vi "Dual XDCR Positioner.vi"(5 "Debug Mode?":bool, 6 "Initial Setup Complete":bool=TRUE, 7 "Main Digitizer":T1=enum."NI Digitizer", 8 "error in (no error)":errorcluster, 9 "Location":T2=enum."WCM Rotation", 10 "Dual XDCR Settings In":T3 {"XDCR Settings"."UT340 Controls"."Low Pass Filter (MHz)" min=-6 max=60 step=1; "XDCR Settings"."UT340 Controls"."High Pass Filter (MHz)" min=1 max=20 step=1; "XDCR Settings"."UT340 Controls"."Rep Rate (Hz)" min=20 step=1; "XDCR Settings"."UT340 Controls"."Pulse Width (ns)" min=100.0 max=250.0 step=2.0; "XDCR Settings"."UT340 Controls"."Voltage" min=100 max=250 step=2; "XDCR Settings"."UT340 Controls"."PC Gain (dB)" min=2 max=72; "XDCR Settings"."UT340 Controls"."PE Gain (dB)" min=-6 max=60 step=1; "XDCR Settings"."JSR Complete"."JSR Trigger Settings"."PRF (Hz)" items=["100 Hz"=0.1, "200 Hz"=0.2, "400 Hz"=0.4, "600 Hz"=0.6, "800 Hz"=0.8, "1000 Hz"=1.0, "1250 Hz"=1.25, "1500 Hz"=1.5, "1750 Hz"=1.75, "2000 Hz"=2.0, "2500 Hz"=2.5, "3000 Hz"=3.0, "3500 Hz"=3.5, "4000 Hz"=4.0, "4500 Hz"=4.5, "5000 Hz"=5.0]; "XDCR Settings"."JSR Complete"."JSR Trigger Settings"."Trigger Source" items=["Internal", "External"]; "XDCR Settings"."JSR Complete"."JSR Trigger Settings"."External Trigger Limit" items=["No Limit", "5 kHz"]; "XDCR Settings"."JSR Complete"."JSR Receive Settings"."Gain (dB)" min=-13 max=66 step=1; "XDCR Settings"."JSR Complete"."JSR Receive Settings"."Low Pass Filter" items=["5 MHz"=5, "10 MHz"=10, "15 MHz"=15, "22.5 MHz"=22, "35 MHz"=35, "50 MHz"=50]; "XDCR Settings"."JSR Complete"."JSR Receive Settings"."High Pass Filter" items=["DC"=0, "1 MHz"=1000, "2.5 MHz"=2500, "5 MHz"=5000, "7.5 MHz"=7500, "12.5 MHz"=12500]; "XDCR Settings"."JSR Complete"."JSR Receive Settings"."Receiver Mode" items=["Echo", "Through"]; "XDCR Settings"."JSR Complete"."JSR Pulse Settings"."Pulser Voltage (V)" items=["100"=100, "125"=125, "150"=150, "175"=175, "200"=200, "225"=225, "250"=250, "275"=275, "300"=300, "325"=325, "350"=350, "375"=375, "400"=400, "425"=425, "450"=450, "475"=475]; "XDCR Settings"."JSR Complete"."JSR Pulse Settings"."Pulser Impedance" items=["High z", "Low z"]; "XDCR Settings"."JSR Complete"."JSR Pulse Settings"."Pulse Energy Level" items=["0 (Minimum)", "1", "2", "3 (Maximum)"]; "XDCR Settings"."JSR Complete"."JSR Pulse Settings"."Damping" items=["331 Ohms"=331, "198 Ohms"=198, "142 Ohms"=142, "110 Ohms"=110, "92 Ohms"=92, "77 Ohms"=77, "67 Ohms"=67, "59 Ohms"=59, "52 Ohms"=52, "47 Ohms"=47, "43 Ohms"=43, "39 Ohms"=39, "37 Ohms"=37, "34 Ohms"=34, "32 Ohms"=32, "30 Ohms"=30]; "XDCR Settings"."Panametrics Settings"."FINE ATTENUATION" items=["00.0", "00.5", "01.0", "01.5", "02.0", "02.5", "03.0", "03.5", "04.0", "04.5", "05.0", "05.5", "06.0", "06.5", "07.0", "07.5", "08.0", "08.5", "09.0", "09.5", "10.0", "10.5", "11.0", "11.5", "12.0", "12.5", "13.0", "13.5", "14.0", "14.5", "15.0", "15.5"]; "XDCR Settings"."Panametrics Settings"."COARSE ATTENUATION" items=["00.0", "10.0", "20.0", "30.0", "40.0", "50.0"]; "XDCR Settings"."Panametrics Settings"."GAIN (db)" items=["26.0", "40.0", "54.0"]; "XDCR Settings"."Panametrics Settings"."PRF (KHz)" items=["XREMT", "EXBNC", "0.200", "0.500", "1.000", "2.000", "5.000", "10.00", "20.00"]; "XDCR Settings"."Panametrics Settings"."MODE" items=["P/ E", "THRU", "RPP", "EXT_PLSR"]; "XDCR Settings"."Panametrics Settings"."LP FILT (MHz)" items=["20", "50", "100", "200"]; "XDCR Settings"."Panametrics Settings"."HP FILT (KHz)" items=["1", "1000", "3000", "10000"]; "XDCR Settings"."Panametrics Settings"."DAMPING (Ohm)" items=["7", "10", "16", "20", "26", "30", "40", "50"]; "XDCR Settings"."Panametrics Settings"."ENERGY (uJ)" items=["1", "2", "4", "8", "16", "32"]; "XDCR Settings"."Daxsonics Settings"."Freq (MHz)" items=["4"=4, "5"=5, "6"=6, "8"=8, "10"=10, "12"=12, "14"=14, "15"=15, "16"=16, "17"=17, "18"=18, "20"=20, "25"=25, "30"=30, "35"=35, "40"=40, "45"=45, "50"=50]; "XDCR Settings"."Daxsonics Settings"."Voltage (V)" items=["0"=0, "5"=5, "10"=10, "15"=15, "20"=20, "25"=25, "30"=30, "35"=35, "40"=40, "45"=45, "50"=50, "55"=55, "60"=60, "65"=65, "70"=70, "75"=75, "80"=80, "85"=85, "90"=90, "95"=95, "100"=100, "110"=110, "120"=120, "130"=130, "140"=140, "150"=150, "160"=160, "170"=170, "180"=180, "190"=190]; "XDCR Settings"."Daxsonics Settings"."Gain (dB)" items=["22"=22, "25"=25, "28"=28, "31"=31, "34"=34, "37"=37, "40"=40, "43"=43, "46"=46, "49"=49, "52"=52, "55"=55, "58"=58, "61"=61, "64"=64, "67"=67]; "XDCR Settings"."Digitizer Settings"."Additional dig delay (ms)" format="%.2f"; "XDCR Settings"."Digitizer Settings"."Time scale per Div" items=["100 ns"=0.1, "200 ns"=0.2, "500 ns"=0.5, "1 micros"=1.0, "2 micros"=2.0, "5 micros"=5.0, "10 micros"=10.0, "20 micros"=20.0, "50 micros"=50.0, "100 micros"=100.0, "200 micros"=200.0, "500 micros"=500.0, "1 ms"=1000.0, "2 ms"=2000.0, "5 ms"=5000.0, "10 ms"=10000.0, "20 ms"=20000.0, "50 ms"=50000.0, "100 ms"=100000.0, "200 ms"=200000.0]; "XDCR Settings"."Digitizer Settings"."RF data Sampling"."rf points per line" min=1; "XDCR Settings"."Digitizer Settings"."RF data Sampling"."Ref Delay (ms)" format="%.2f"}, 11 "Motion Settings":T23={"No Motion?"=FALSE, "Motion System"=enum."NI 735x", "Motion Bd ID"=1, "Motion Profile"="SMAC1", "# Axis"=1, "Reverse Z axis?"=TRUE, "SMAC Axis"=0, "scan pair"=enum."y-(x) scan", "RT fps"=6.0, "Steps per mm"=[1000, 1000, 1000, 1000], "Motor Parameters"={"velocity ct/s"=[10000.0, 10000.0, 10000.0, 50000.0], "accel ct/s^2"=[50000.0, 50000.0, 50000.0, 200000.0]}, "One Way Scan"=FALSE, "Reverse One Way Scan"=FALSE, "Global Position (mm)"=[], "Plane"=0, "Distance between\nscan lines (um)"=0.0, "Distance between\nscan planes (um)"=0.0, "number of scan planes"=1, "Total steps in line"=0, "Xtra plane\ndistance  (um)"=100, "Xtra planes "=1, "Add Axis"=FALSE, "overshoot cts"=200, "BKPT Shift"=0, "Scan Start Time (ms)"=0, "ESP VISA"="GPIB::1::INSTR", "3rd Axis"=1, "GL Ref Out"=refnum, "Galil Address"=""} {"3rd Axis" items=["x", "y", "z", "w"]; "Xtra planes" min=1; "Xtra plane\ndistance  (um)" min=0; "Distance between\nscan planes (um)" format="%.2f"; "Distance between\nscan lines (um)" format="%.2f"; "SMAC Axis" items=["None"=0, "Axis 1"=1, "Axis 2"=2, "Axis 3"=3, "Axis 4"=4, "Axis 5"=5, "Axis 6"=6, "Axis 7"=7, "Axis 8"=8, "Vector Space 1"=17, "Vector Space 2"=18, "Vector Space 3"=19, "Vector Space 4"=20]; "Motion Bd ID" min=1 max=32 step=1}) -> (0 "error out":errorcluster, 1 "Switch T/R":u32, 2 "Dual XDCR Settings":T3 {"XDCR Settings"."UT340 Controls"."Low Pass Filter (MHz)" min=-6 max=60 step=1; "XDCR Settings"."UT340 Controls"."High Pass Filter (MHz)" min=1 max=20 step=1; "XDCR Settings"."UT340 Controls"."Rep Rate (Hz)" min=20 step=1; "XDCR Settings"."UT340 Controls"."Pulse Width (ns)" min=100.0 max=250.0 step=2.0; "XDCR Settings"."UT340 Controls"."Voltage" min=100 max=250 step=2; "XDCR Settings"."UT340 Controls"."PC Gain (dB)" min=2 max=72; "XDCR Settings"."UT340 Controls"."PE Gain (dB)" min=-6 max=60 step=1; "XDCR Settings"."JSR Complete"."JSR Trigger Settings"."PRF (Hz)" items=["100 Hz"=0.1, "200 Hz"=0.2, "400 Hz"=0.4, "600 Hz"=0.6, "800 Hz"=0.8, "1000 Hz"=1.0, "1250 Hz"=1.25, "1500 Hz"=1.5, "1750 Hz"=1.75, "2000 Hz"=2.0, "2500 Hz"=2.5, "3000 Hz"=3.0, "3500 Hz"=3.5, "4000 Hz"=4.0, "4500 Hz"=4.5, "5000 Hz"=5.0]; "XDCR Settings"."JSR Complete"."JSR Trigger Settings"."Trigger Source" items=["Internal", "External"]; "XDCR Settings"."JSR Complete"."JSR Trigger Settings"."External Trigger Limit" items=["No Limit", "5 kHz"]; "XDCR Settings"."JSR Complete"."JSR Receive Settings"."Gain (dB)" min=-13 max=66 step=1; "XDCR Settings"."JSR Complete"."JSR Receive Settings"."Low Pass Filter" items=["5 MHz"=5, "10 MHz"=10, "15 MHz"=15, "22.5 MHz"=22, "35 MHz"=35, "50 MHz"=50]; "XDCR Settings"."JSR Complete"."JSR Receive Settings"."High Pass Filter" items=["DC"=0, "1 MHz"=1000, "2.5 MHz"=2500, "5 MHz"=5000, "7.5 MHz"=7500, "12.5 MHz"=12500]; "XDCR Settings"."JSR Complete"."JSR Receive Settings"."Receiver Mode" items=["Echo", "Through"]; "XDCR Settings"."JSR Complete"."JSR Pulse Settings"."Pulser Voltage (V)" items=["100"=100, "125"=125, "150"=150, "175"=175, "200"=200, "225"=225, "250"=250, "275"=275, "300"=300, "325"=325, "350"=350, "375"=375, "400"=400, "425"=425, "450"=450, "475"=475]; "XDCR Settings"."JSR Complete"."JSR Pulse Settings"."Pulser Impedance" items=["High z", "Low z"]; "XDCR Settings"."JSR Complete"."JSR Pulse Settings"."Pulse Energy Level" items=["0 (Minimum)", "1", "2", "3 (Maximum)"]; "XDCR Settings"."JSR Complete"."JSR Pulse Settings"."Damping" items=["331 Ohms"=331, "198 Ohms"=198, "142 Ohms"=142, "110 Ohms"=110, "92 Ohms"=92, "77 Ohms"=77, "67 Ohms"=67, "59 Ohms"=59, "52 Ohms"=52, "47 Ohms"=47, "43 Ohms"=43, "39 Ohms"=39, "37 Ohms"=37, "34 Ohms"=34, "32 Ohms"=32, "30 Ohms"=30]; "XDCR Settings"."Panametrics Settings"."FINE ATTENUATION" items=["00.0", "00.5", "01.0", "01.5", "02.0", "02.5", "03.0", "03.5", "04.0", "04.5", "05.0", "05.5", "06.0", "06.5", "07.0", "07.5", "08.0", "08.5", "09.0", "09.5", "10.0", "10.5", "11.0", "11.5", "12.0", "12.5", "13.0", "13.5", "14.0", "14.5", "15.0", "15.5"]; "XDCR Settings"."Panametrics Settings"."COARSE ATTENUATION" items=["00.0", "10.0", "20.0", "30.0", "40.0", "50.0"]; "XDCR Settings"."Panametrics Settings"."GAIN (db)" items=["26.0", "40.0", "54.0"]; "XDCR Settings"."Panametrics Settings"."PRF (KHz)" items=["XREMT", "EXBNC", "0.200", "0.500", "1.000", "2.000", "5.000", "10.00", "20.00"]; "XDCR Settings"."Panametrics Settings"."MODE" items=["P/ E", "THRU", "RPP", "EXT_PLSR"]; "XDCR Settings"."Panametrics Settings"."LP FILT (MHz)" items=["20", "50", "100", "200"]; "XDCR Settings"."Panametrics Settings"."HP FILT (KHz)" items=["1", "1000", "3000", "10000"]; "XDCR Settings"."Panametrics Settings"."DAMPING (Ohm)" items=["7", "10", "16", "20", "26", "30", "40", "50"]; "XDCR Settings"."Panametrics Settings"."ENERGY (uJ)" items=["1", "2", "4", "8", "16", "32"]; "XDCR Settings"."Daxsonics Settings"."Freq (MHz)" items=["4"=4, "5"=5, "6"=6, "8"=8, "10"=10, "12"=12, "14"=14, "15"=15, "16"=16, "17"=17, "18"=18, "20"=20, "25"=25, "30"=30, "35"=35, "40"=40, "45"=45, "50"=50]; "XDCR Settings"."Daxsonics Settings"."Voltage (V)" items=["0"=0, "5"=5, "10"=10, "15"=15, "20"=20, "25"=25, "30"=30, "35"=35, "40"=40, "45"=45, "50"=50, "55"=55, "60"=60, "65"=65, "70"=70, "75"=75, "80"=80, "85"=85, "90"=90, "95"=95, "100"=100, "110"=110, "120"=120, "130"=130, "140"=140, "150"=150, "160"=160, "170"=170, "180"=180, "190"=190]; "XDCR Settings"."Daxsonics Settings"."Gain (dB)" items=["22"=22, "25"=25, "28"=28, "31"=31, "34"=34, "37"=37, "40"=40, "43"=43, "46"=46, "49"=49, "52"=52, "55"=55, "58"=58, "61"=61, "64"=64, "67"=67]; "XDCR Settings"."Digitizer Settings"."Additional dig delay (ms)" format="%.2f"; "XDCR Settings"."Digitizer Settings"."Time scale per Div" items=["100 ns"=0.1, "200 ns"=0.2, "500 ns"=0.5, "1 micros"=1.0, "2 micros"=2.0, "5 micros"=5.0, "10 micros"=10.0, "20 micros"=20.0, "50 micros"=50.0, "100 micros"=100.0, "200 micros"=200.0, "500 micros"=500.0, "1 ms"=1000.0, "2 ms"=2000.0, "5 ms"=5000.0, "10 ms"=10000.0, "20 ms"=20000.0, "50 ms"=50000.0, "100 ms"=100000.0, "200 ms"=200000.0]; "XDCR Settings"."Digitizer Settings"."RF data Sampling"."rf points per line" min=1; "XDCR Settings"."Digitizer Settings"."RF data Sampling"."Ref Delay (ms)" format="%.2f"}, 3 "Motion Settings Out":T23={"No Motion?"=FALSE, "Motion System"=enum."NI 735x", "Motion Bd ID"=1, "Motion Profile"="SMAC1", "# Axis"=1, "Reverse Z axis?"=TRUE, "SMAC Axis"=0, "scan pair"=enum."y-(x) scan", "RT fps"=6.0, "Steps per mm"=[1000, 1000, 1000, 1000], "Motor Parameters"={"velocity ct/s"=[10000.0, 10000.0, 10000.0, 50000.0], "accel ct/s^2"=[50000.0, 50000.0, 50000.0, 200000.0]}, "One Way Scan"=FALSE, "Reverse One Way Scan"=FALSE, "Global Position (mm)"=[], "Plane"=0, "Distance between\nscan lines (um)"=0.0, "Distance between\nscan planes (um)"=0.0, "number of scan planes"=1, "Total steps in line"=0, "Xtra plane\ndistance  (um)"=100, "Xtra planes "=1, "Add Axis"=FALSE, "overshoot cts"=200, "BKPT Shift"=0, "Scan Start Time (ms)"=0, "ESP VISA"="GPIB::1::INSTR", "3rd Axis"=1, "GL Ref Out"=refnum, "Galil Address"=""} {"3rd Axis" items=["x", "y", "z", "w"]; "Xtra planes" min=1; "Xtra plane\ndistance  (um)" min=0; "Distance between\nscan planes (um)" format="%.2f"; "Distance between\nscan lines (um)" format="%.2f"; "SMAC Axis" items=["None"=0, "Axis 1"=1, "Axis 2"=2, "Axis 3"=3, "Axis 4"=4, "Axis 5"=5, "Axis 6"=6, "Axis 7"=7, "Axis 8"=8, "Vector Space 1"=17, "Vector Space 2"=18, "Vector Space 3"=19, "Vector Space 4"=20]; "Motion Bd ID" min=1 max=32 step=1}, 4 "Default Selected?":bool)   [LabVIEW 2022 SP3]
uses:
  Motion Controllers/NI_controller/-NI_MotionRoutines/MotionParameters.ctl
  Motion Controllers/NI_controller/-NI_MotionRoutines/MotionSys.ctl
  Motion Controllers/-MotionRoutines/ScanAxis.ctl
  Motion Controllers/-MotionRoutines/3rdAxis.ctl
  Dual XDCR Complete Settings.ctl
  XDCRSettings.ctl
  Pulsers/Daxsonics/-DaxSubroutines/Dax_Control_Cluster.ctl
  Pulsers/Panametrics/Pana5900.ctl
  Pulsers/JSR/Controls/JSR Complete.ctl
  Pulsers/JSR/Controls/JSR Pulse.ctl
  Pulsers/JSR/Controls/Damping.ctl
  Pulsers/JSR/Controls/Energy.ctl
  Pulsers/JSR/Controls/Z.ctl
  Pulsers/JSR/Controls/Volt.ctl
  Pulsers/JSR/Controls/JSR Recieve.ctl
  Pulsers/JSR/Controls/Mode.ctl
  Pulsers/JSR/Controls/HPF.ctl
  Pulsers/JSR/Controls/LPF.ctl
  Pulsers/JSR/Controls/Gain.ctl
  Pulsers/JSR/Controls/JSR Trigger.ctl
  Pulsers/JSR/Controls/Trig Limit.ctl
  Pulsers/JSR/Controls/Trig Source.ctl
  Pulsers/JSR/Controls/PRF.ctl
  Pulsers/UTEX/Controls/UTEX Controls.ctl
  -ScanSystem/Controls/location.ctl
  Digitizers/-DigitizerRoutines/Digitizer.ctl
  <vilib>/Motion/FlexMotion/CustomControls/CustomControls.llb/AxisOrVectorSpaceControl To Control.flx
panel:
  out "Abort":bool
  # "1-D and 2-D B scan settings"
  # "1-D and 2-D B scan settings"
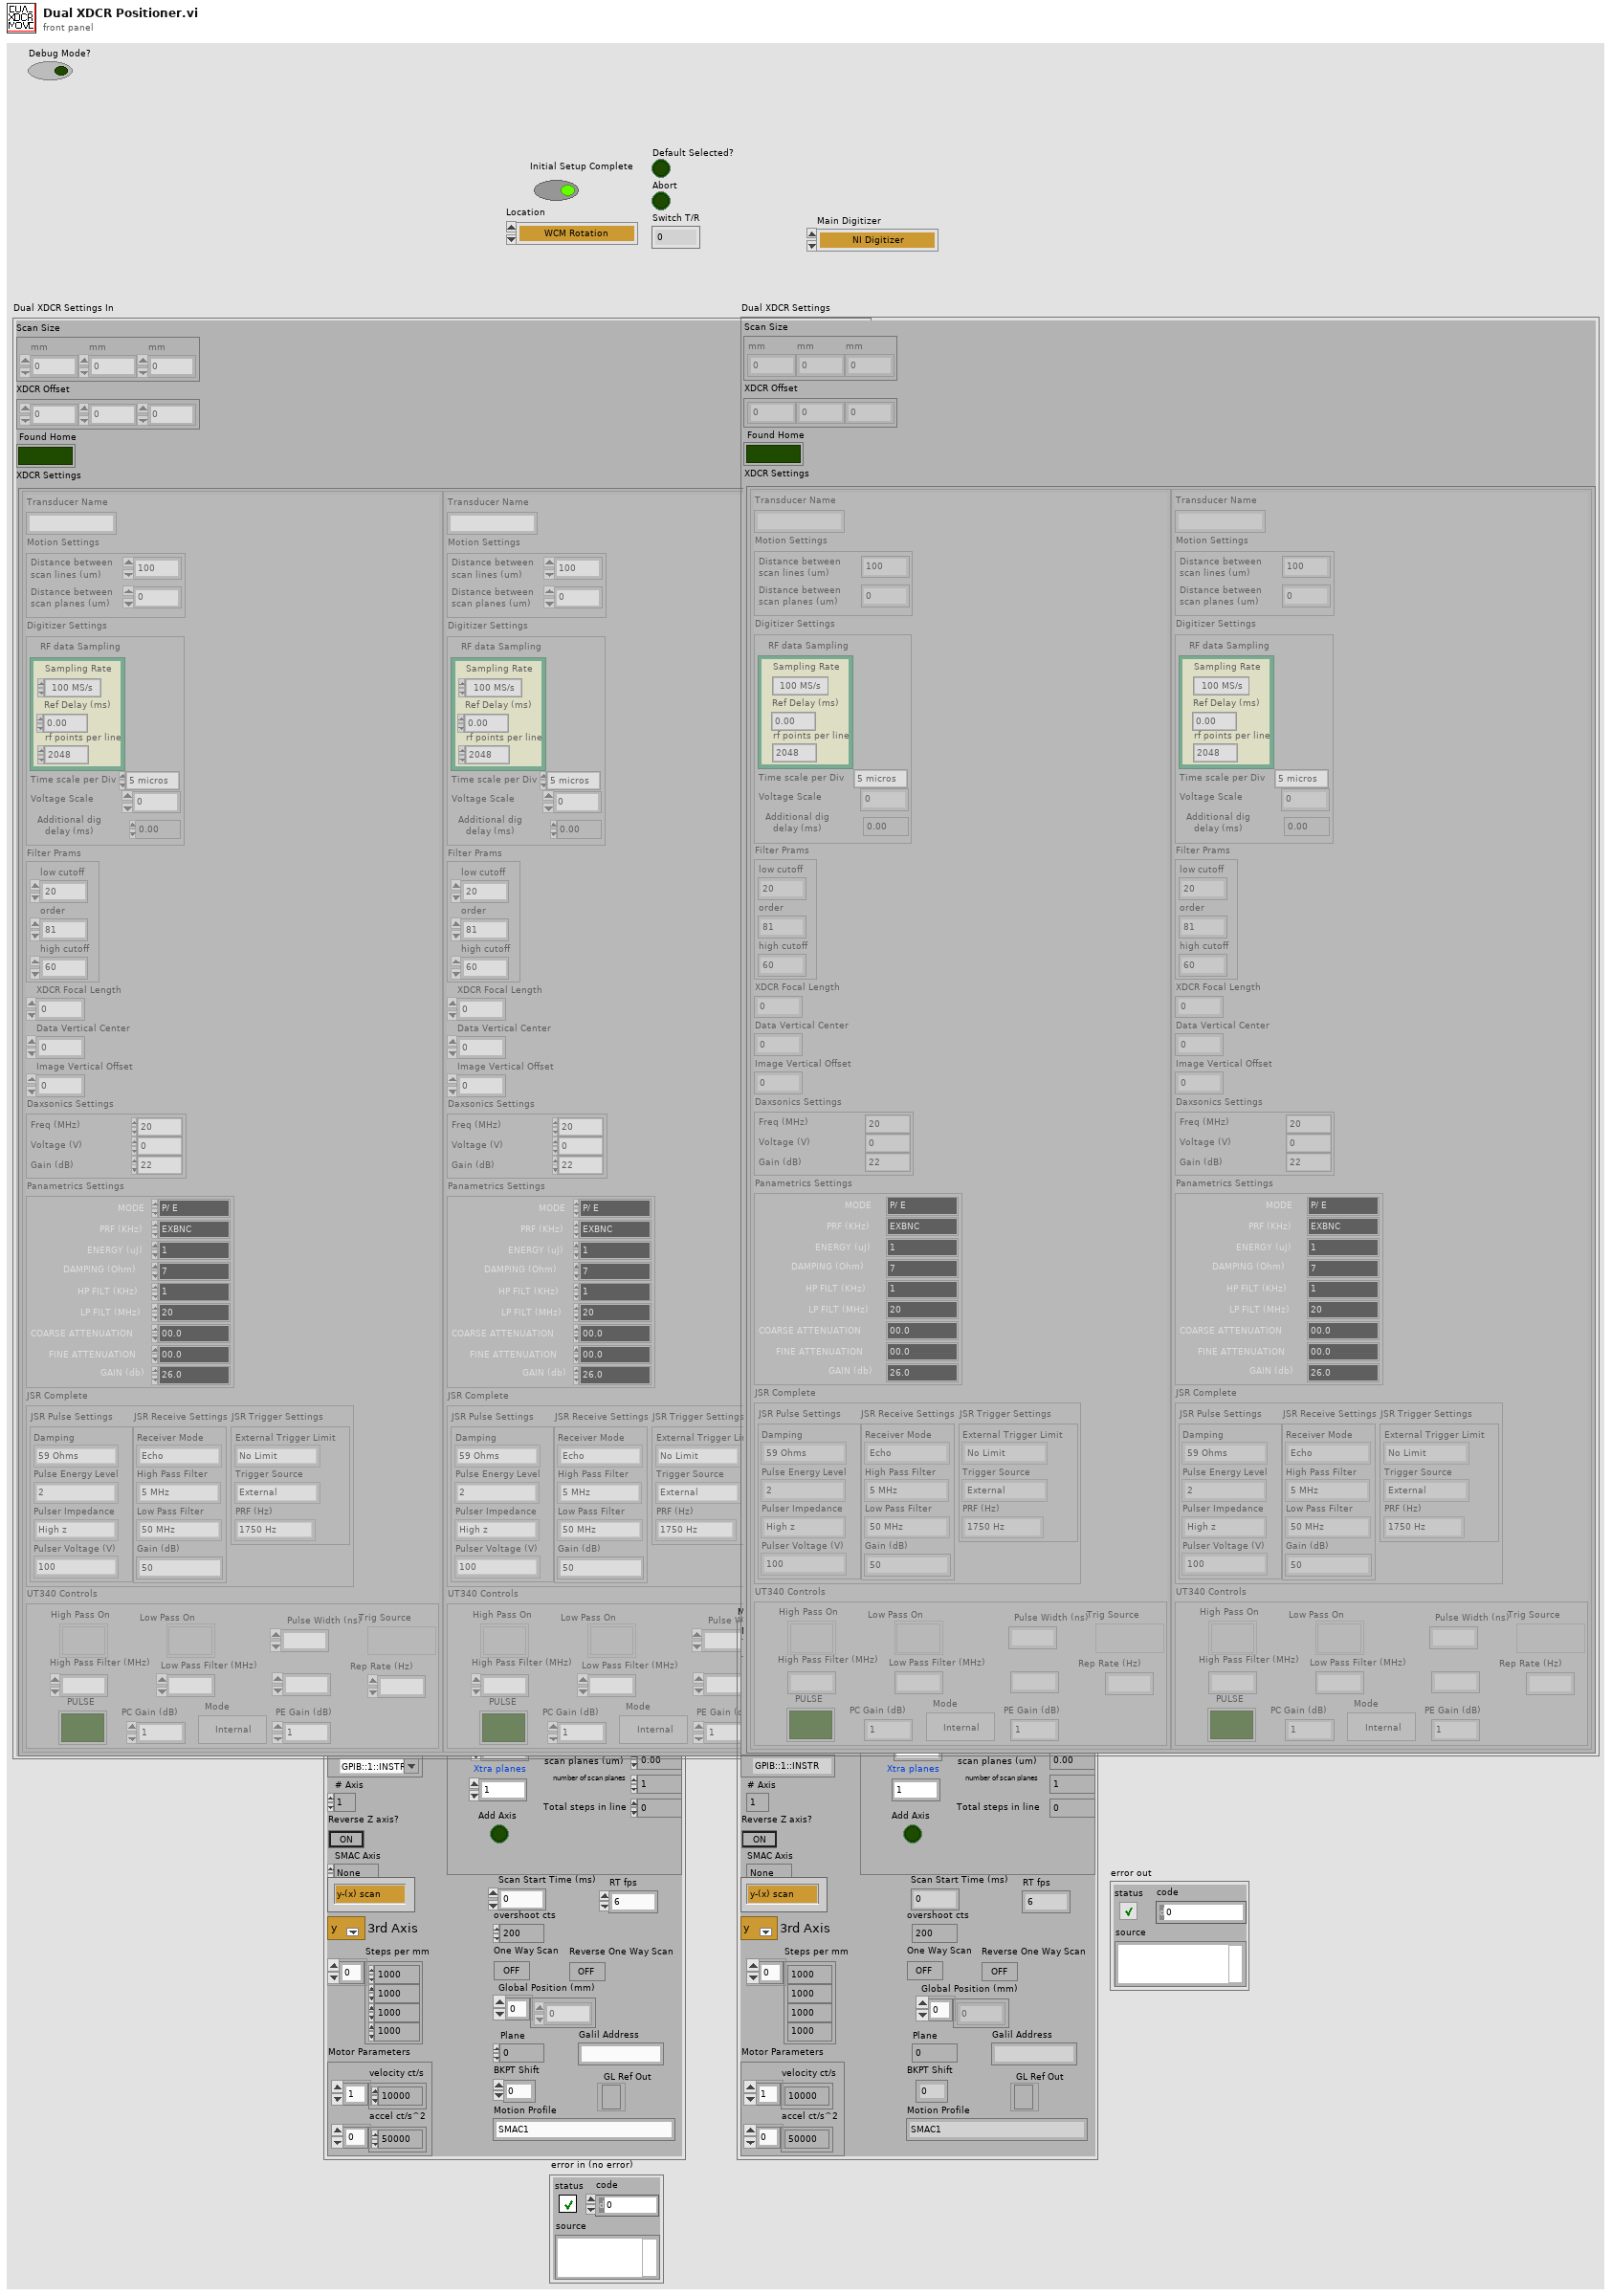
[diagram p1: front panel]
types:
  T1 = typedef "Digitizer.ctl" = enum16{"Acqiris Digitizer", "NI Digitizer", "LeCroy", "GaGe", "AlazarTech", "No Digitizer", "Teledyne"}
  T2 = typedef "location.ctl" = enum16{"Automatic", "WCM Main", "Hawaii", "Columbia MM3000", "Columbia  NI System", "NYU", "RRI 2", "UHI Allen", "CUMC RT", "Chiba", "Stony Brook", "WCM Microscopy", "WCM Aeoretch", "WCM Optics Lab", "WCM Main 2Axis", "WCM Rotation", "WCM SAM SMAC", "SERI GP"}
  T3 = typedef "Dual XDCR Complete Settings.ctl" = cluster{"Scan Size":dbl[], "XDCR Offset":dbl[], "Found Home":bool, "XDCR Settings":T4[]}
  T4 = typedef "XDCRSettings.ctl" = cluster{"Transducer Name":string, "Motion Settings":cluster{"Distance between\nscan lines (um)":sgl, "Distance between\nscan planes (um)":sgl}, "Digitizer Settings":cluster{"RF data Sampling":cluster{"Sampling Rate":dbl, "Ref Delay (ms)":dbl, "rf points per line":i32}, "Time scale per Div":dbl, "Voltage Scale":dbl, "Additional dig delay (ms)":dbl}, "Filter Prams":cluster{"low cutoff":i32, "order":i32, "high cutoff":i32}, "XDCR Focal Length":dbl, "Data Vertical Center":dbl, "Image Vertical Offset":dbl, "Daxsonics Settings":T5, "Panametrics Settings":T6, "JSR Complete":T7, "UT340 Controls":T22}
  T5 = typedef "Dax_Control_Cluster.ctl" = cluster{"Freq (MHz) ":u16, "Voltage (V)":u16, "Gain (dB)":u16}
  T6 = typedef "Pana5900.ctl" = cluster{"ENERGY (uJ)":u16, "DAMPING (Ohm)":u16, "HP FILT (KHz) ":u16, "LP FILT (MHz)":u16, "MODE":u16, "PRF (KHz)":u16, "GAIN (db)":u16, "COARSE ATTENUATION":u16, "FINE ATTENUATION":u16}
  T7 = typedef "JSR Complete.ctl" = cluster{"JSR Pulse Settings":T8, "JSR Receive Settings":T13, "JSR Trigger Settings":T18}
  T8 = typedef "JSR Pulse.ctl" = cluster{"Damping":T9, "Pulse Energy Level":T10, "Pulser Impedance":T11, "Pulser Voltage (V)":T12}
  T9 = typedef "Damping.ctl" = i16
  T10 = typedef "Energy.ctl" = u16
  T11 = typedef "Z.ctl" = u16
  T12 = typedef "Volt.ctl" = i16
  T13 = typedef "JSR Recieve.ctl" = cluster{"Receiver Mode":T14, "High Pass Filter":T15, "Low Pass Filter":T16, "Gain (dB)":T17}
  T14 = typedef "Mode.ctl" = i8
  T15 = typedef "HPF.ctl" = u16
  T16 = typedef "LPF.ctl" = u16
  T17 = typedef "Gain.ctl" = i8
  T18 = typedef "JSR Trigger.ctl" = cluster{"External Trigger Limit":T19, "Trigger Source":T20, "PRF (Hz)":T21}
  T19 = typedef "Trig Limit.ctl" = i8
  T20 = typedef "Trig Source.ctl" = i8
  T21 = typedef "PRF.ctl" = dbl
  T22 = typedef "UTEX Controls.ctl" = cluster{"High Pass On":bool, "High Pass Filter (MHz)":i16, "Low Pass On":bool, "Low Pass Filter (MHz)":i16, "PE Gain (dB)":i16, "Voltage":i16, "Pulse Width (ns)":dbl, "Mode":bool, "PC Gain (dB)":i16, "Trig Source":bool, "Rep Rate (Hz)":i16, "PULSE":bool}
  T23 = typedef "MotionParameters.ctl" = cluster{"No Motion?":bool, "Motion System":T24, "Motion Bd ID":u8, "Motion Profile":string, "# Axis":i8, "Reverse Z axis?":bool, "SMAC Axis":u16, "scan pair":T25, "RT fps":sgl, "Steps per mm":i32[], "Motor Parameters":cluster{"velocity ct/s":dbl[], "accel ct/s^2":dbl[]}, "One Way Scan":bool, "Reverse One Way Scan":bool, "Global Position (mm)":dbl[], "Plane":i32, "Distance between\nscan lines (um)":sgl, "Distance between\nscan planes (um)":sgl, "number of scan planes":i32, "Total steps in line":i32, "Xtra plane\ndistance  (um)":i32, "Xtra planes ":i32, "Add Axis":bool, "overshoot cts":i32, "BKPT Shift":i32, "Scan Start Time (ms)":u32, "ESP VISA":refnum<visa-resource-name>, "3rd Axis":T26, "GL Ref Out":refnum<k7>, "Galil Address":string}
  T24 = typedef "MotionSys.ctl" = enum16{"MM3000", "NI 735x", "Newport ESP", "No Motion Card", "Galil"}
  T25 = typedef "ScanAxis.ctl" = enum16{"y-(x) scan", "x-(y) scan", "z-(x) scan", "z-(y) scan", "y-(z) scan", "x-(z) scan", "w-(x) scan", "w-(y) scan", "w-(z) scan", "x-(w) scan", "y-(w) scan", "z-(w) scan"}
  T26 = typedef "3rdAxis.ctl" = u16
  T27 = enum16{"Left Button", "Center Button", "Right Button", "Window Close"}
  T28 = cluster{"1":bool, "2":bool, "3":bool, "4":bool, "5":bool, "6":bool, "7":bool, "8":bool}
  T29 = enum16{"Absolute Position", "Relative Position", "Velocity", "Relative to Cap Pos", "Modulus Position", "Absolute Contouring", "Relative Contouring"}
  T30 = enum16{"Home", "Index", "Center", "Forward Limit", "Reverse Limit", "Run Sequence"}
  T31 = typedef "AxisOrVectorSpaceControl To Control.flx" = u16
  T32 = typedef "Bd Id Out" = u8
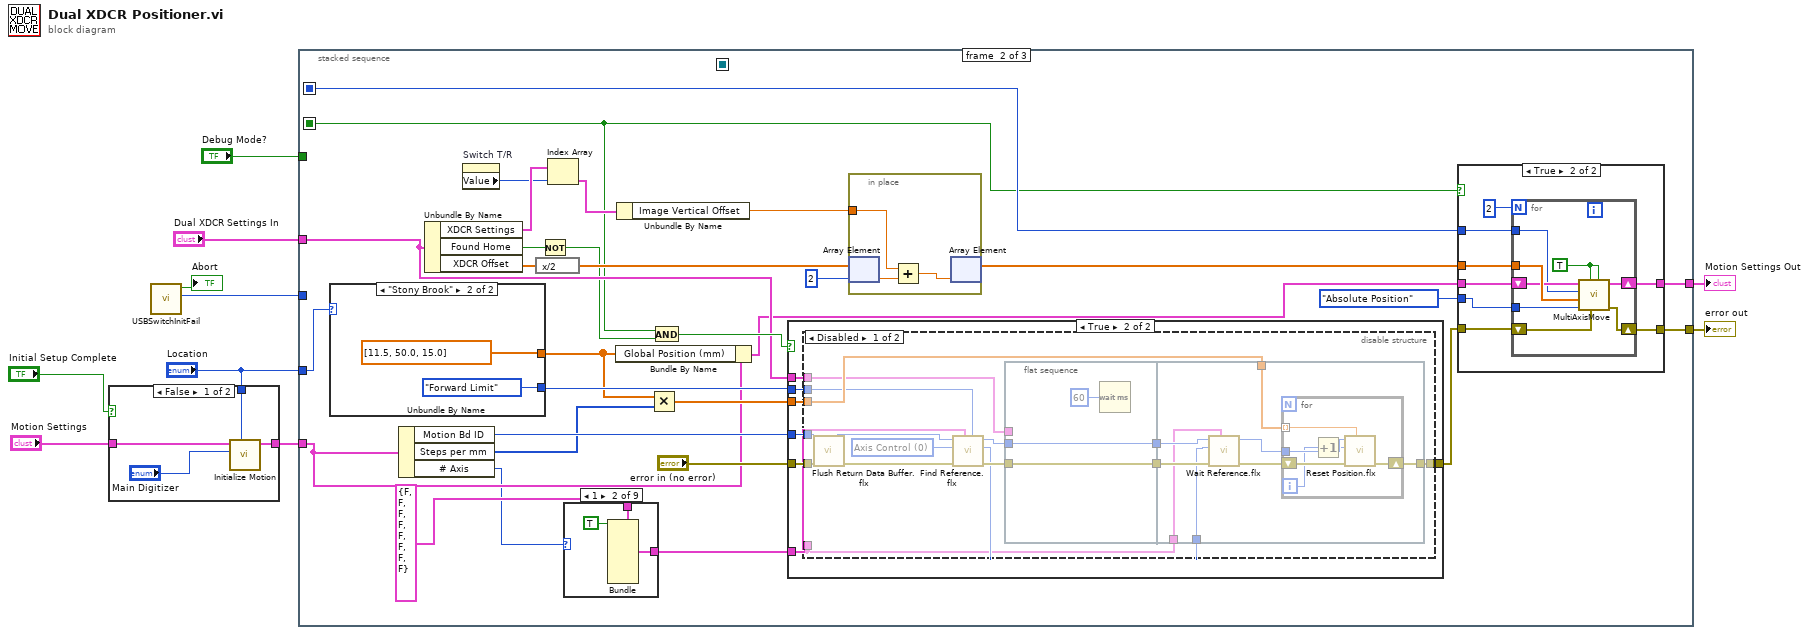
[diagram p0: block diagram]
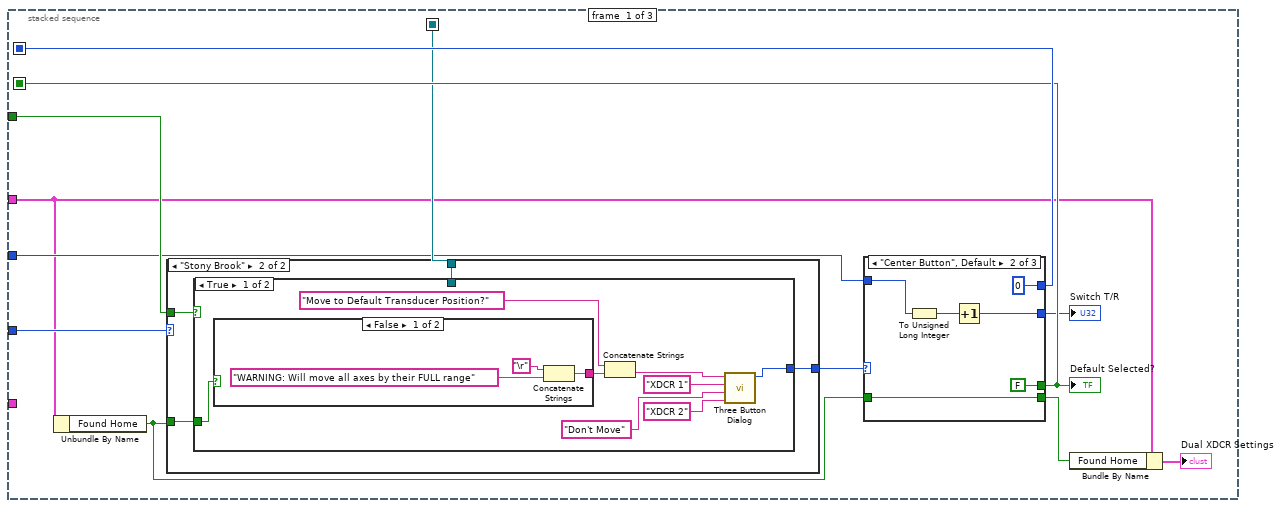
[diagram p3: hidden frame]
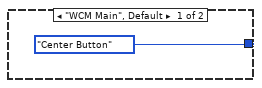
[diagram p4: hidden frame]
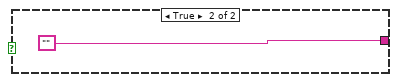
[diagram p5: hidden frame]
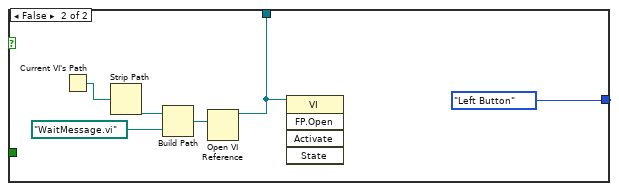
[diagram p6: hidden frame]
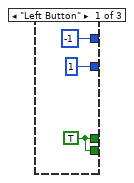
[diagram p7: hidden frame]
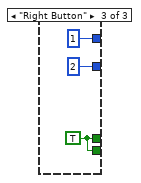
[diagram p8: hidden frame]
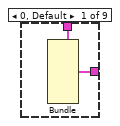
[diagram p9: hidden frame]
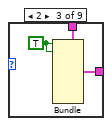
[diagram p10: hidden frame]
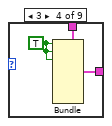
[diagram p11: hidden frame]
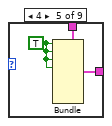
[diagram p12: hidden frame]
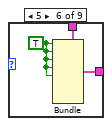
[diagram p13: hidden frame]
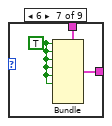
[diagram p14: hidden frame]
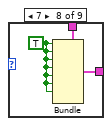
[diagram p15: hidden frame]
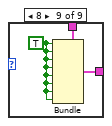
[diagram p16: hidden frame]
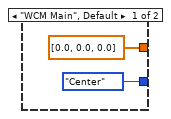
[diagram p20: hidden frame]
diagram:
  n1 = case shown="False" "Initial Setup Complete" {
    tunnel: "Motion Settings" -> [w14 w15]
    tunnel: [w13 w15] -> w6
    tunnel: "Location" -> [w11 _]
    frame False {
      n2 = call "Initialize Motion.vi"("Location"=w11, "Main Digitizer"="Main Digitizer", "Motion Settings In"=w14) -> ("Motion Settings"=w13:T23)  [unwired: 6 in, 2 out]
    }
    frame True {
    }
  }
  n3 = call "USBSwitchInitFail.vi"() -> ("Transducer"=w2:enum16{"Transducer 1", "Transducer 2"}, "Abort"=→"Abort":bool)  [unwired: 10 in]
  n4 = stacked-sequence {
    seq-local: [w24 _ _] -> [_ w84 w184]
    seq-local: [w23 _ _] -> [_ w67 _]
    seq-local: [w19 _ _] -> [_ _ w185]
    tunnel: "Dual XDCR Settings In" -> [w16 w81 _]
    tunnel: [_ w83 _] -> w9
    tunnel: [_ w82 _] -> w8
    tunnel: w6 -> [_ w79 _]
    tunnel: "Location" -> [w22 w69 w186]
    tunnel: "Debug Mode?" -> [w18 _ _]
    tunnel: w2 -> [w17 _ _]
    frame #0 {
      n5 = Unbundle By Name(w16) -> ("Found Home"=w21:bool)
      n6 = case shown="\"Stony Brook\"" w22 {
        tunnel: [T27."Center Button" ("Which Button?") w32] -> w27
        tunnel: w21 -> [_ w30]
        tunnel: [_ w31] -> w19
        tunnel: w18 -> [_ w29]
        frame "WCM Main", Default {
        }
        frame "Stony Brook" {
          n7 = case shown="True" w29 {
            tunnel: [w34 T27."Left Button" ("Which Button?")] -> w32
            tunnel: [_ w49] -> w31
            tunnel: w30 -> [w33 _]
            frame True {
              n8 = case shown="False" w33 {
                tunnel: [w41 "" ("message")] -> w35
                frame False {
                  n9 = Concatenate Strings("\r", "WARNING: Will move all axes by their FULL range" ("message")) -> (w41:string)
                }
                frame True {
                }
              }
              n10 = Concatenate Strings("Move to Default Transducer Position?" ("message"), w35) -> (w37:string)
              n11 = call <vilib>:"Three Button Dialog.vi"("Right Button Text (\"Cancel\")"="XDCR 2" ("Right Button Text (\"Cancel\")"), "Center Button Text (\"No\")"="Don't Move" ("F button name (\"Cancel\")"), "Left Button Text (\"Yes\")"="XDCR 1" ("T button name (\"OK\")"), "message"=w37) -> ("Which Button?"=w34:T27)  [unwired: 7 in]
            }
            frame False {
              n12 = Current VI's Path() -> (path=w47:path)
              n13 = Strip Path(path=w47) -> (stripped path=w45:path)  [unwired: 1 out]
              n14 = Build Path(base path=w45, name or relative path=path "WaitMessage.vi" ("vi path")) -> (appended path=w48:path)
              n15 = Open VI Reference(vi path=w48) -> (vi reference=w49:refnum<vi>)  [unwired: 5 in, 1 out]
              n16 = invoke class="VI" method="FP.Open"(reference=w49) -> ()  [unwired: 4 in, 5 out]
            }
          }
        }
      }
      n17 = case shown="\"Center Button\", Default" w27 {
        tunnel: [w51 FALSE w60] -> w23
        tunnel: [-1 ("Move Polarity") 0 ("Move Polarity") 1 ("Move Polarity")] -> w24
        tunnel: [u32 1 ("Switch T/R") w57 u32 2 ("Switch T/R")] -> w20
        tunnel: [w51 w56 w60] -> w26
        tunnel: w21 -> [_ w56 _]
        tunnel: w17 -> [_ w54 _]
        frame "Left Button" {
          w51 = TRUE ("Found Home")
        }
        frame "Center Button", Default {
          n18 = To Unsigned Long Integer(number=w54) -> (unsigned 32bit integer=w55:u32)
          n19 = Increment(x=w55) -> (x+1=w57:u32)
        }
        frame "Right Button" {
          w60 = TRUE ("Found Home")
        }
      }
      "Switch T/R" <- w20
      "Default Selected?" <- w23
      n20 = Bundle By Name(cluster=w16, "Found Home"=w26) -> (→"Dual XDCR Settings":T3)
    }
    frame #1 {
      n21 = case shown="\"Stony Brook\"" w69 {
        tunnel: [T30."Center" ("Search Type") T30."Forward Limit" ("Search Type")] -> w89
        tunnel: [dbl[] [0.0, 0.0, 0.0] ("Primary Reset Position (0)") dbl[] [11.5, 50.0, 15.0] ("Primary Reset Position (0)")] -> w78
        frame "WCM Main", Default {
        }
        frame "Stony Brook" {
        }
      }
      n22 = Unbundle By Name(w79) -> ("Motion Bd ID"=w88:u8, "Steps per mm"=w77:i32[], "# Axis"=w63:i8)
      n23 = Unbundle By Name(w81) -> ("XDCR Settings"=w76:T4[], "Found Home"=w87:bool, "XDCR Offset"=w85:dbl[])
      n24 = property on="Switch T/R" class="DigNum (strict)"() -> ("Value"=w75:u32)  [unwired: 2 in, 2 out]
      n25 = expression code="x/2"(w85) -> (w73:dbl[])
      n26 = Not(x=w87) -> (.not. x?=w66:bool)
      n27 = Index Array(array=w76, index=w75) -> (element=w74:T4)
      n28 = case shown="1" w63 {
        tunnel: [w94 w97 w100 w103 w106 w109 w112 w115 w118] -> w65
        tunnel: T28 {"1"=FALSE, "2"=FALSE, "3"=FALSE, "4"=FALSE, "5"=FALSE, "6"=FALSE, "7"=FALSE, "8"=FALSE} ("Axis/VS Map (Disabled)") -> [w93 w96 w99 w102 w105 w108 w111 w114 w117]
        frame 0, Default {
          n29 = Bundle(cluster=w93) -> (w94:T28)  [unwired: 8 in]
        }
        frame 1 {
          n30 = Bundle(cluster=w96, "1"=TRUE) -> (w97:T28)  [unwired: 7 in]
        }
        frame 2 {
          w98 = TRUE ("1")
          n31 = Bundle(cluster=w99, "1"=w98, "2"=w98) -> (w100:T28)  [unwired: 6 in]
        }
        frame 3 {
          w101 = TRUE ("1")
          n32 = Bundle(cluster=w102, "1"=w101, "2"=w101, "3"=w101) -> (w103:T28)  [unwired: 5 in]
        }
        frame 4 {
          w104 = TRUE ("1")
          n33 = Bundle(cluster=w105, "1"=w104, "2"=w104, "3"=w104, "4"=w104) -> (w106:T28)  [unwired: 4 in]
        }
        frame 5 {
          w107 = TRUE ("1")
          n34 = Bundle(cluster=w108, "1"=w107, "2"=w107, "3"=w107, "4"=w107, "5"=w107) -> (w109:T28)  [unwired: 3 in]
        }
        frame 6 {
          w110 = TRUE ("1")
          n35 = Bundle(cluster=w111, "1"=w110, "2"=w110, "3"=w110, "4"=w110, "5"=w110, "6"=w110) -> (w112:T28)  [unwired: 2 in]
        }
        frame 7 {
          w113 = TRUE ("1")
          n36 = Bundle(cluster=w114, "1"=w113, "2"=w113, "3"=w113, "4"=w113, "5"=w113, "6"=w113, "7"=w113) -> (w115:T28)  [unwired: 1 in]
        }
        frame 8 {
          w116 = TRUE ("1")
          n37 = Bundle(cluster=w117, "1"=w116, "2"=w116, "3"=w116, "4"=w116, "5"=w116, "6"=w116, "7"=w116, "8"=w116) -> (w118:T28)
        }
      }
      n38 = Bundle By Name(cluster=w79, "Global Position (mm)"=w78) -> (w80:T23)
      n39 = Unbundle By Name(w74) -> ("Image Vertical Offset"=w71:dbl)
      n40 = Multiply(x=w78, y=w77) -> (x*y=w92:dbl[])
      n41 = And(x=w67, y=w66) -> (x .and. y?=w91:bool)
      n42 = case shown="True" w91 {
        tunnel: "error in (no error)" -> [w140 w143]
        tunnel: w92 -> [_ w147]
        tunnel: w89 -> [_ w146]
        tunnel: w88 -> [_ w144]
        tunnel: w81 -> [_ w145]
        tunnel: [w140 w142] -> w68
        tunnel: w65 -> [_ w141]
        frame False {
        }
        frame True {
          n43 = disable-structure shown="Disabled" {
            disable-tunnel: w147 -> [w158 _]
            disable-tunnel: w146 -> [w157 _]
            disable-tunnel: w145 -> [w156 _]
            disable-tunnel: w144 -> [w154 _]
            disable-tunnel: w143 -> [w152 _]
            disable-tunnel: [w150 _] -> w142
            disable-tunnel: w141 -> [w148 _]
            frame Disabled {
              w155 = T31 0 items=["Axis Control"=0, "Axis 1"=1, "Axis 2"=2, "Axis 3"=3, "Axis 4"=4, "Axis 5"=5, "Axis 6"=6, "Axis 7"=7, "Axis 8"=8, "Vector Space Control"=16, "Vector Space 1"=17, "Vector Space 2"=18, "Vector Space 3"=19, "Vector Space 4"=20] ("Axis or Vector Space")
              n44 = call <vilib>:"Flush Return Data Buffer.flx"("error in (no error)"=w152, "Board ID"=w154) -> ("error out"=w151:errorcluster, "Bd ID Out"=w153:T32)  [unwired: 5 in]
              n45 = call <vilib>:"Find Reference.flx"("Search Type"=w157, "Axis/VS Map (Disabled)"=w148, "error in (no error)"=w151, "Axis or Vector Space"=w155, "Board ID"=w153) -> ("error out"=w159:errorcluster, "Axis or Vector Space Output"=w149:T31, "Bd ID Out"=w160:T32)  [unwired: 4 in]
              n46 = flat-sequence {
                tunnel: w159 -> [w164]
                tunnel: w160 -> [w165]
                tunnel: [w165] -> w162
                tunnel: [w164] -> w161
                tunnel: w156 -> [_]
                tunnel: w162 -> [w173]
                tunnel: w161 -> [w172]
                tunnel: w158 -> [w170]
                tunnel: [w169] -> w150
                tunnel: w149 -> [w167]
                tunnel: w148 -> [w166]
                frame #0 {
                  n47 = Wait (ms)(milliseconds to wait=u32 60) -> ()  [unwired: 1 out]
                }
                frame #1 {
                  n48 = call <vilib>:"Wait Reference.flx"("Axis/VS Map (Disabled)"=w166, "error in (no error)"=w172, "Axis or Vector Space"=w167, "Board ID"=w173) -> ("error out"=w168:errorcluster, "Bd ID Out"=w171:T32)  [unwired: 4 in, 2 out]
                  n49 = for {
                    tunnel: w171 -> [w179]
                    tunnel: w170 -> [w178] mode=indexing
                    shift-right: [w177] -> w169
                    shift-left: w168 -> [w176]
                    i -> [w175]
                    n50 = Increment(x=w175) -> (x+1=w174:i32)
                    n51 = call <vilib>:"Reset Position.flx"("Primary Reset Position (0)"=w178, "error in (no error)"=w176, "Axis"=w174, "Board ID"=w179) -> ("error out"=w177:errorcluster)  [unwired: 1 in, 4 out]
                  }
                }
              }
            }
            frame Enabled {
            }
          }
        }
      }
      n52 = in-place {
        in-place-border: w71 -> [w119]
        n53 = in-place-array #1(w73, 2) -> (w121:dbl)
        n54 = Add(x=w119, y=w121) -> (x+y=w120:dbl)
        n55 = in-place-array #1(w120) -> (w72:dbl[])  [unwired: 1 out]
      }
      n56 = case shown="True" w67 {
        tunnel: [w122 w131] -> w82
        tunnel: [w123 w130] -> w83
        tunnel: w72 -> [_ w129]
        tunnel: T29."Absolute Position" ("Position Mode (Absolute)") -> [_ w128]
        tunnel: w80 -> [w123 w127]
        tunnel: w84 -> [_ w126]
        tunnel: w68 -> [w122 w124]
        frame False {
        }
        frame True {
          n57 = for {
            N: 2 -> [_]
            tunnel: w129 -> [w136]
            tunnel: w128 -> [w135]
            tunnel: w126 -> [w133]
            shift-right: [w139] -> w131
            shift-left: w124 -> [w137]
            shift-right: [w138] -> w130
            shift-left: w127 -> [w134]
            w132 = TRUE ("Wait For Move Complete")
            n58 = call "MultiAxisMove.vi"("Find Location"=w132, "error in"=w137, "Wait For Move Complete"=w132, "Position Mode (Rel)"=w135, "Distance to move (mm)"=w136, "Move Polarity"=w133, "Motion Settings"=w134) -> ("error out"=w139:errorcluster, "Motion Settings Out"=w138:T23)  [unwired: 2 in, 1 out]
          }
        }
      }
    }
    frame #2 {
      n59 = case shown="\"Stony Brook\"" w186 {
        tunnel: w185 -> [_ w189]
        tunnel: w184 -> [_ w188]
        frame "WCM Main", Default {
        }
        frame "Stony Brook" {
          n60 = Not Equal To 0?(x=w188) -> (x != 0?=w187:bool)
          n61 = case shown="True" w187 {
            tunnel: w189 -> [_ w193]
            frame False {
            }
            frame True {
              n62 = call "WaitMessage.vi"("stop"=TRUE) -> ("error in (no error) 2"=w192:errorcluster)  [unwired: 10 in]
              n63 = invoke class="VI" method="FP.Close"(reference=w193, error in=w192) -> (error out=w190:errorcluster)  [unwired: 1 in, 2 out]
              n64 = property on="error out" class="Clust (strict)"("Value"=w190) -> ()  [unwired: 2 in, 2 out]
            }
          }
        }
      }
    }
  }
  "error out" <- w8
  "Motion Settings Out" <- w9
